vi "Get Data.vi"(8 "error in (no error)":errorcluster, 10 "Name":string, 11 "Dictionary in":refnum<class "Dictionary.lvclass">) -> (0 "error out":errorcluster, 2 "Value":variant, 3 "Dictionary out":refnum<class "Dictionary.lvclass">)   [LabVIEW 2014, in "bmlv.lvlib" / "Dictionary.lvclass"]
uses:
  Dictionary.lvclass
  Dictionary.lvclass/Dictionary.ctl
  Read Dict.vi
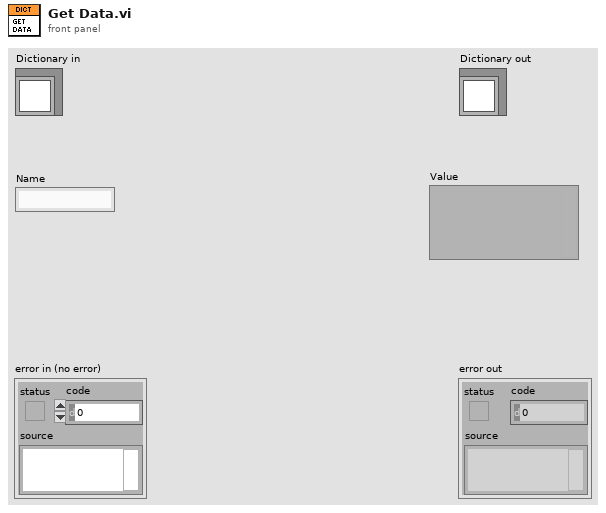
[diagram p1: front panel]
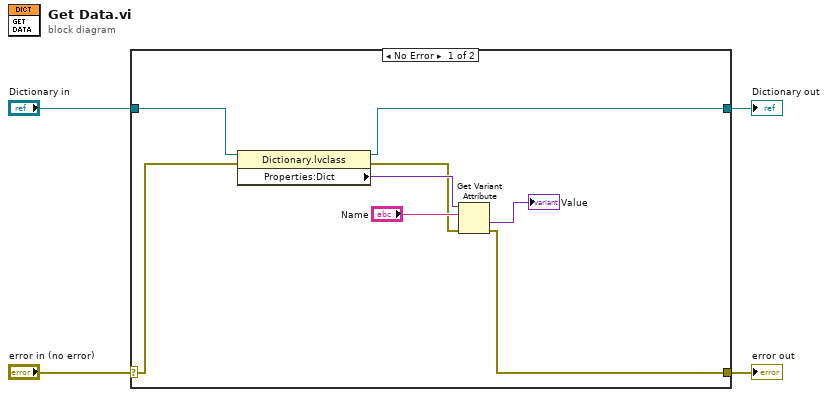
[diagram p0: block diagram]
diagram:
  n1 = case shown="No Error" "error in (no error)" {
    selector: "error in (no error)" -> [w8 w14]
    tunnel: [w5 w14] -> w3
    tunnel: [w9 w13] -> w1
    tunnel: "Dictionary in" -> [w12 w13]
    frame No Error {
      n2 = property class="Dictionary.lvclass"(reference=w12, error in=w8) -> (reference out=w9:refnum<class "Dictionary.lvclass">, error out=w7:errorcluster, "Properties:Dict"=w11:variant)
      n3 = Get Variant Attribute(Variant=w11, name="Name", error in=w7) -> (value=→"Value":variant, error out=w5:errorcluster)  [unwired: 1 in, 2 out]
    }
    frame Error {
    }
  }
  "error out" <- w3
  "Dictionary out" <- w1
